vi "波形图与闸门取值.vi"(5 "错误输入":errorcluster, 7 "波形数据":dbl[][](array[numeric]), 8 "闸门 4":cluster{"起点":u8, "宽度":u8, "高度":u8}={"起点"=64, "宽度"=10, "高度"=44} {"高度" scale=0.0..50.0; "宽度" scale=0.0..10.0; "起点" scale=0.0..150.0}, 9 "闸门 3":cluster{"起点":u8, "宽度":u8, "高度":u8}={"起点"=64, "宽度"=10, "高度"=44} {"高度" scale=0.0..50.0; "宽度" scale=0.0..10.0; "起点" scale=0.0..150.0}, 10 "闸门 2":cluster{"起点":u8, "宽度":u8, "高度":u8}={"起点"=64, "宽度"=10, "高度"=44} {"高度" scale=0.0..50.0; "宽度" scale=0.0..10.0; "起点" scale=0.0..150.0}, 11 "闸门":cluster{"起点":u8, "宽度":u8, "高度":u8}={"起点"=64, "宽度"=10, "高度"=44} {"高度" scale=0.0..50.0; "宽度" scale=0.0..10.0; "起点" scale=0.0..150.0}) -> (0 "错误输出":errorcluster, 1 "XY图":cluster{"波形数据":dbl[], "波形数据":dbl[]}[](graph), 2 "Y":dbl[](array[numeric]), 3 "X":dbl[](array[numeric]))   [LabVIEW 2018]
panel:
  in  "转置的数组":dbl[][](array[numeric])
  in  "间隔":dbl=0.04 format="%#_13g"
  # "测试用数组\n4096X2"
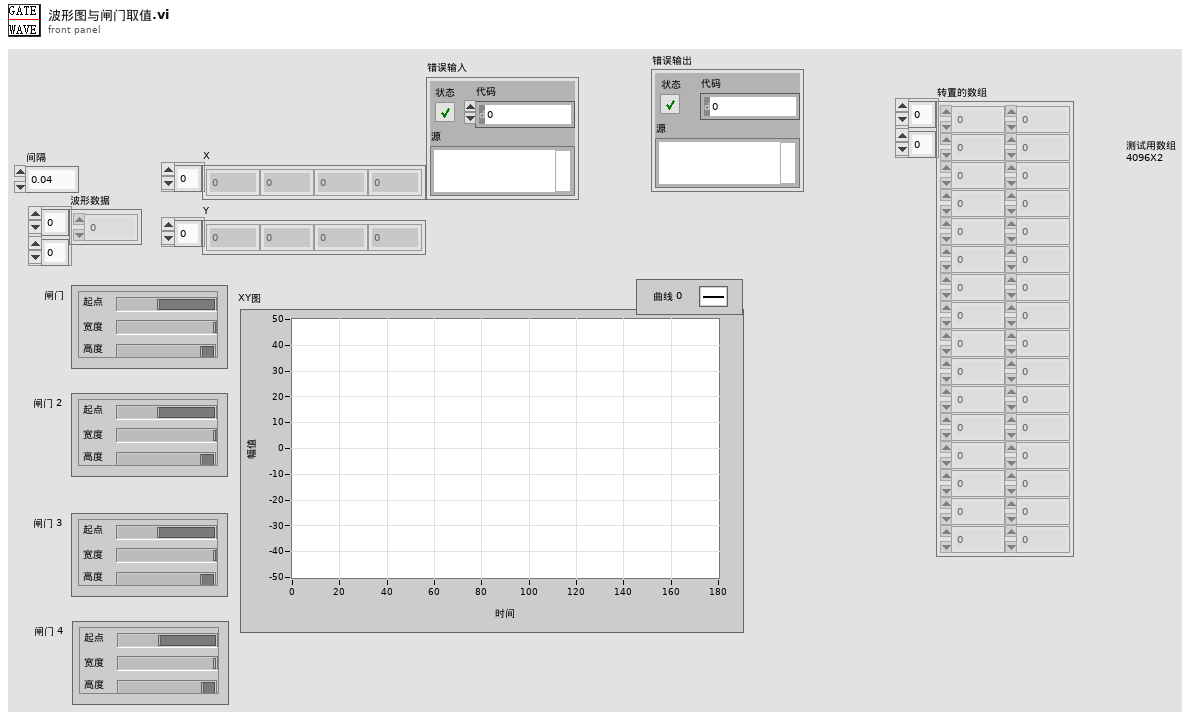
[diagram p1: front panel]
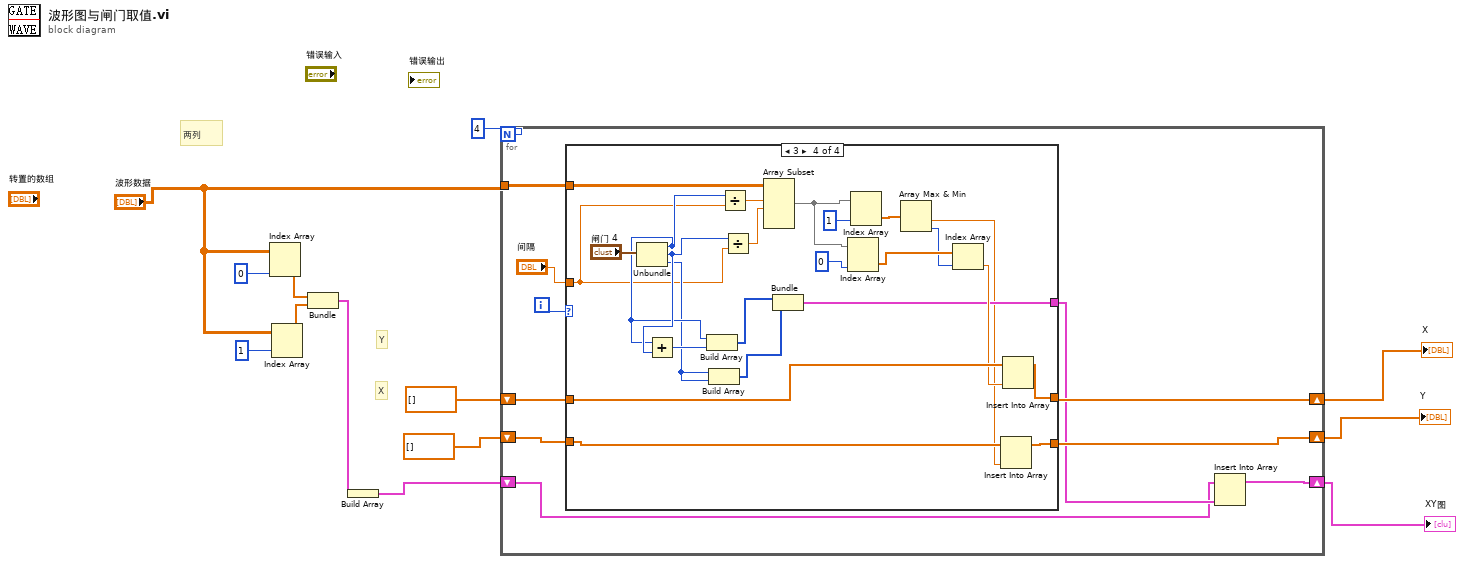
[diagram p0: block diagram]
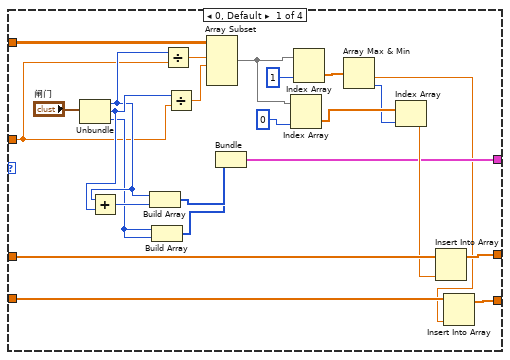
[diagram p2: hidden frame]
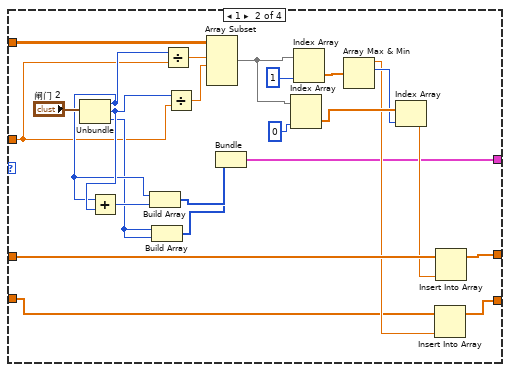
[diagram p3: hidden frame]
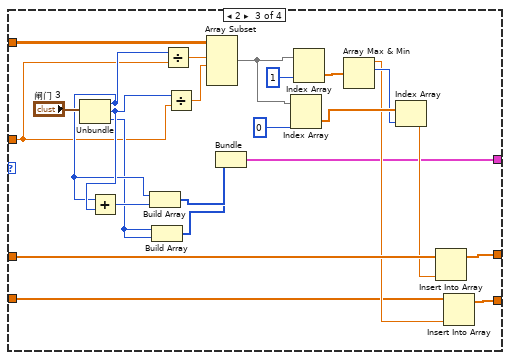
[diagram p4: hidden frame]
diagram:
  # "两列"
  # "Y"
  # "X"
  n1 = Index Array(array="波形数据", index (col)=0 ("索引 (行)")) -> (element=w8:dbl[])  [unwired: 1 in]
  n2 = Index Array(array="波形数据", index (col)=1 ("索引 (行)")) -> (element=w7:dbl[])  [unwired: 1 in]
  n3 = Bundle("波形数据"=w8, "波形数据"=w7) -> (w6:cluster{"波形数据":dbl[], "波形数据":dbl[]})  [unwired: 1 in]
  n4 = Build Array(w6) -> (w3:cluster{"波形数据":dbl[], "波形数据":dbl[]}[])
  n5 = for {
    N: 4 -> [_]
    tunnel: "波形数据" -> [w22]
    shift-right: [w20] -> w10
    shift-left: dbl[] [] ("子数组") -> [w21]
    shift-right: [w18] -> w9
    shift-left: dbl[] [] ("子数组") -> [w19]
    shift-right: [w14] -> w2
    shift-left: w3 -> [w15]
    i -> [w23]
    n6 = case shown="3" w23 {
      tunnel: w22 -> [w44 w68 w92 w116]
      tunnel: w21 -> [w40 w63 w87 w112]
      tunnel: [w38 w61 w85 w110] -> w20
      tunnel: w19 -> [w37 w59 w83 w109]
      tunnel: [w36 w58 w82 w108] -> w18
      tunnel: [w29 w51 w75 w101] -> w16
      tunnel: "间隔" -> [w26 w48 w72 w98]
      frame 0, Default {
        n7 = Unbundle("闸门") -> ("起点"=w33:u8, "宽度"=w35:u8, "高度"=w32:u8)
        n8 = Add(x=w33, y=w35) -> (x+y=w34:u8)
        n9 = Build Array(w33, w34) -> (w31:u8[])
        n10 = Build Array(w32, w32) -> (w30:u8[])
        n11 = Divide(x=w33, y=w26) -> (x/y=w46:dbl)
        n12 = Divide(x=w35, y=w26) -> (x/y=w45:dbl)
        n13 = Array Subset(array=w44, index (row)=w46, length (row)=w45) -> (w43:dbl[][])  [unwired: 2 in]
        n14 = Bundle(w31, w30) -> (w29:cluster{u8[], u8[]})  [unwired: 1 in]
        n15 = Index Array(array=w43, index (col)=0 ("索引")) -> (element=w41:dbl[])  [unwired: 1 in]
        n16 = Index Array(array=w43, index (col)=1 ("索引")) -> (element=w42:dbl[])  [unwired: 1 in]
        n17 = Array Max & Min(array=w42) -> (min value=w25:dbl, min index (indices)=w24:i32)  [unwired: 2 out]
        n18 = Index Array(array=w41, index=w24) -> (element=w39:dbl)
        n19 = Insert Into Array(array=w40, new element=w39) -> (w38:dbl[])  [unwired: 1 in]
        n20 = Insert Into Array(array=w37, new element=w25) -> (w36:dbl[])  [unwired: 1 in]
      }
      frame 1 {
        n21 = Unbundle("闸门 2") -> ("起点"=w55:u8, "宽度"=w57:u8, "高度"=w54:u8)
        n22 = Add(x=w55, y=w57) -> (x+y=w56:u8)
        n23 = Build Array(w55, w56) -> (w53:u8[])
        n24 = Build Array(w54, w54) -> (w52:u8[])
        n25 = Divide(x=w55, y=w48) -> (x/y=w70:dbl)
        n26 = Divide(x=w57, y=w48) -> (x/y=w69:dbl)
        n27 = Array Subset(array=w68, index (row)=w70, length (row)=w69) -> (w67:dbl[][])  [unwired: 2 in]
        n28 = Bundle(w53, w52) -> (w51:cluster{u8[], u8[]})  [unwired: 1 in]
        n29 = Index Array(array=w67, index (col)=0 ("索引")) -> (element=w65:dbl[])  [unwired: 1 in]
        n30 = Index Array(array=w67, index (col)=1 ("索引")) -> (element=w66:dbl[])  [unwired: 1 in]
        n31 = Array Max & Min(array=w66) -> (max value=w60:dbl, max index (indices)=w64:i32)  [unwired: 2 out]
        n32 = Index Array(array=w65, index=w64) -> (element=w62:dbl)
        n33 = Insert Into Array(array=w59, new element=w60) -> (w58:dbl[])  [unwired: 1 in]
        n34 = Insert Into Array(array=w63, new element=w62) -> (w61:dbl[])  [unwired: 1 in]
      }
      frame 2 {
        n35 = Unbundle("闸门 3") -> ("起点"=w79:u8, "宽度"=w81:u8, "高度"=w78:u8)
        n36 = Add(x=w79, y=w81) -> (x+y=w80:u8)
        n37 = Build Array(w79, w80) -> (w77:u8[])
        n38 = Build Array(w78, w78) -> (w76:u8[])
        n39 = Divide(x=w79, y=w72) -> (x/y=w94:dbl)
        n40 = Divide(x=w81, y=w72) -> (x/y=w93:dbl)
        n41 = Array Subset(array=w92, index (row)=w94, length (row)=w93) -> (w91:dbl[][])  [unwired: 2 in]
        n42 = Bundle(w77, w76) -> (w75:cluster{u8[], u8[]})  [unwired: 1 in]
        n43 = Index Array(array=w91, index (col)=0 ("索引")) -> (element=w89:dbl[])  [unwired: 1 in]
        n44 = Index Array(array=w91, index (col)=1 ("索引")) -> (element=w90:dbl[])  [unwired: 1 in]
        n45 = Array Max & Min(array=w90) -> (max value=w84:dbl, max index (indices)=w88:i32)  [unwired: 2 out]
        n46 = Index Array(array=w89, index=w88) -> (element=w86:dbl)
        n47 = Insert Into Array(array=w87, new element=w86) -> (w85:dbl[])  [unwired: 1 in]
        n48 = Insert Into Array(array=w83, new element=w84) -> (w82:dbl[])  [unwired: 1 in]
      }
      frame 3 {
        n49 = Unbundle("闸门 4") -> ("起点"=w105:u8, "宽度"=w107:u8, "高度"=w104:u8)
        n50 = Add(x=w105, y=w107) -> (x+y=w106:u8)
        n51 = Build Array(w105, w106) -> (w103:u8[])
        n52 = Build Array(w104, w104) -> (w102:u8[])
        n53 = Divide(x=w105, y=w98) -> (x/y=w118:dbl)
        n54 = Divide(x=w107, y=w98) -> (x/y=w117:dbl)
        n55 = Array Subset(array=w116, index (row)=w118, length (row)=w117) -> (w115:dbl[][])  [unwired: 2 in]
        n56 = Bundle(w103, w102) -> (w101:cluster{u8[], u8[]})  [unwired: 1 in]
        n57 = Index Array(array=w115, index (col)=0 ("索引")) -> (element=w113:dbl[])  [unwired: 1 in]
        n58 = Index Array(array=w115, index (col)=1 ("索引")) -> (element=w114:dbl[])  [unwired: 1 in]
        n59 = Array Max & Min(array=w114) -> (min value=w97:dbl, min index (indices)=w96:i32)  [unwired: 2 out]
        n60 = Index Array(array=w113, index=w96) -> (element=w111:dbl)
        n61 = Insert Into Array(array=w109, new element=w97) -> (w108:dbl[])  [unwired: 1 in]
        n62 = Insert Into Array(array=w112, new element=w111) -> (w110:dbl[])  [unwired: 1 in]
      }
    }
    n63 = Insert Into Array(array=w15, new element=w16) -> (w14:cluster{"波形数据":dbl[], "波形数据":dbl[]}[])  [unwired: 1 in]
  }
  "X" <- w10
  "Y" <- w9
  "XY图" <- w2
